vi "GetNewPosition.vi"(9 "Direction":T1, 10 "position in":cluster{"row":i32, "col":i32}, 11 "size(s)":i32[](array[numeric])) -> (3 "position out":cluster{"row":i32, "col":i32})   [LabVIEW 2020]
doc: "Takes size of a Board (2D array), a position(row, column) on that Board and a Direction Enum.\nCalculates next position in the provided direction."
uses:
  TypeDef/direction.ctl
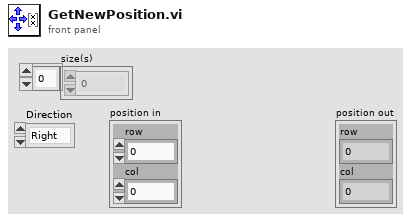
[diagram p1: front panel]
types:
  T1 = typedef "direction.ctl" = enum16{"Right", "Up", "Left", "Down"}
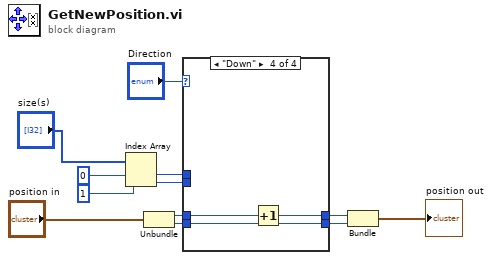
[diagram p0: block diagram]
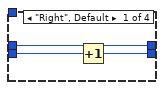
[diagram p2: hidden frame]
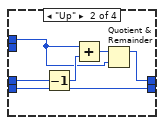
[diagram p3: hidden frame]
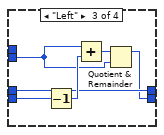
[diagram p4: hidden frame]
diagram:
  n1 = Index Array(array="size(s)", index #1=0 ("index"), index #2=1 ("index")) -> (element #1=w11:i32, element #2=w12:i32)
  n2 = Unbundle("position in") -> ("row"=w7:i32, "col"=w6:i32)
  n3 = case shown="\"Down\"" "Direction" {
    tunnel: w6 -> [w14 w21 w25 w29]
    tunnel: w7 -> [w15 w20 w24 w30]
    tunnel: [w15 w16 w24 w28] -> w4
    tunnel: [w13 w21 w23 w29] -> w3
    tunnel: w11 -> [_ w17 _ _]
    tunnel: w12 -> [_ _ w22 _]
    frame "Right", Default {
      n4 = Increment(x=w14) -> (x+1=w13:i32)
    }
    frame "Up" {
      n5 = Decrement(x=w20) -> (x-1=w18:i32)
      n6 = Add(x=w17, y=w18) -> (x+y=w19:i32)
      n7 = Quotient & Remainder(x=w19, y=w17) -> (x-y*floor(x/y)=w16:i32)  [unwired: 1 out]
    }
    frame "Left" {
      n8 = Decrement(x=w25) -> (x-1=w26:i32)
      n9 = Add(x=w22, y=w26) -> (x+y=w27:i32)
      n10 = Quotient & Remainder(x=w27, y=w22) -> (x-y*floor(x/y)=w23:i32)  [unwired: 1 out]
    }
    frame "Down" {
      n11 = Increment(x=w30) -> (x+1=w28:i32)
    }
  }
  n12 = Bundle("row"=w4, "col"=w3) -> (→"position out":cluster{"row":i32, "col":i32})  [unwired: 1 in]
